vi "test vi.vi"() -> ()   [LabVIEW 2014]
uses:
  Lightning base/Auton Modes.ctl
panel:
  in  "Numeric":i32
  out "Auton Types":T1
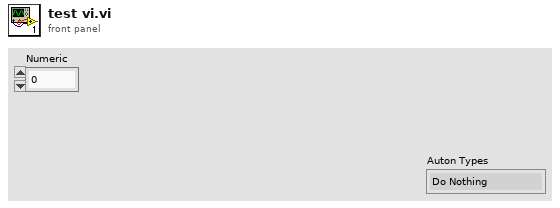
[diagram p1: front panel]
types:
  T1 = typedef "Auton Modes.ctl" = enum16{"Do Nothing", "Move Forward", "Move Forward w/Tote", "Move Forward w/RC", "Gather RC from Step", "3 Tote Auton", "Vision Test", "Strafer"}
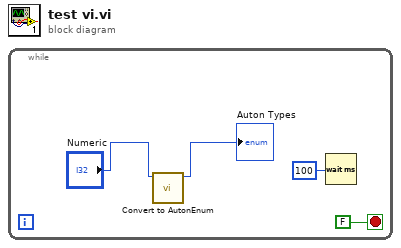
[diagram p0: block diagram]
diagram:
  n1 = while {
    stop <- FALSE stop-if-true
    n2 = call "Convert to AutonEnum.vi"("Auton In"="Numeric") -> ("Auton Out"=→"Auton Types":T1)  [unwired: 10 in]
    n3 = Wait (ms)(milliseconds to wait=u32 100) -> ()  [unwired: 1 out]
  }
